vi "Demo7-Broader_Control_Panel.vi"() -> ()   [LabVIEW 2020]
panel:
  in  "Visualization Tab Control":enum32{"Trace", "Metrics"}(tab)
  out "Diode Trace":waveform(dbl)[](graph)
  out "Reduced Mean Signal, One Point = One Shot":dbl[](graph)
  out "(For your Reference: ) Query Sent to Device":string
  in  "Zero Time":bool
  out "Settable Device Keywords":string[](array[string])
  out "Live Readback Values":string[](array[string])
  in  "Set All":bool
  in  "Set Values\n(Fully empty cells will not be set)":string[](array[string])
  out "Live Responses":string[](array[string])
  out "Non-Settable Device Keywords":string[](array[string])
  in  "IP Address of Remote Device":string="196.254.31.200"
  in  "Disconnect":bool
  # "Diode Demo - General Purpose Control Panel"
  # "General control panel to facilitate setup of diode, setting times, verifying quality of metrics."
  # "VI Instructions\n\n1. Make sure you know the Device IP Address.\n2. From Windows command prompt, confirm ping to IP address.\n3. Type the correct device IP address into this VI.\n3. Run this VI. *Note:* Only one TCP connection to the device's SCPI-like server can run at a time.\n4. When finished, disconnect safely from the device via the \"Disconnect\" toggle button. (Not the Abort button).\n\nCreated by Scott Feister on July 19, 2022.\nUpdated back panel details July 28, 2022."
  # "1. Resets the trigger count to zero.\n2. Transmits this system's current time."
  # "Settings *ARE NOT SAVED TO DEVICE* and are lost on device reset! Write them down!"
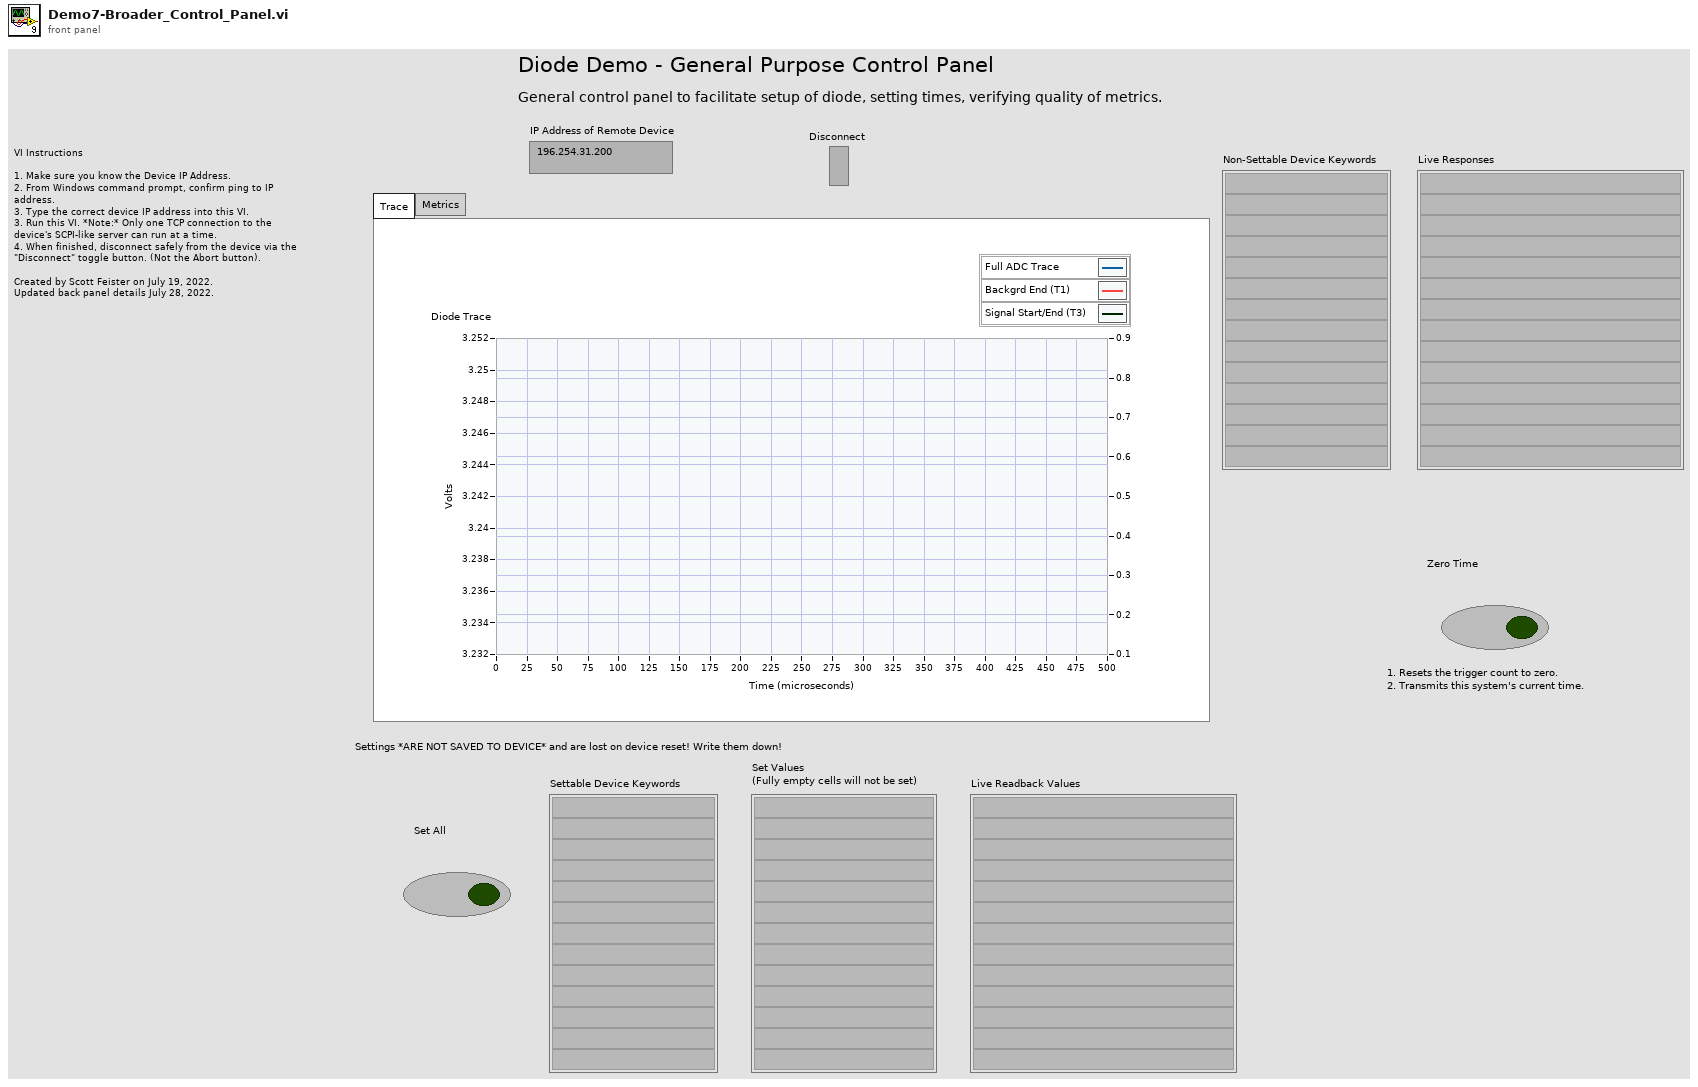
[diagram p1: front panel]
types:
  T1 = typedef "DDAQ-Keyword.ctl" = cluster{"Keyword":string, "Gettable":bool, "Settable":bool, "Is Array":bool, "Data Type":string, "Description":string}
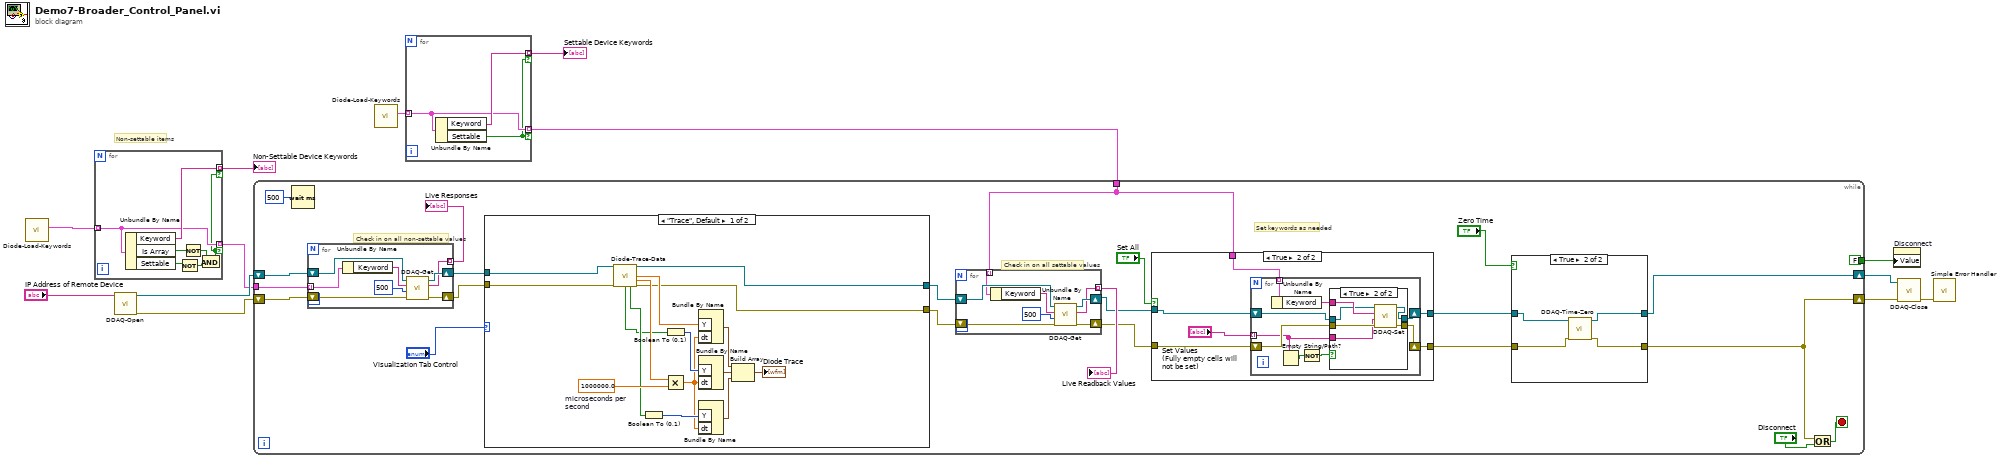
[diagram p0: block diagram]
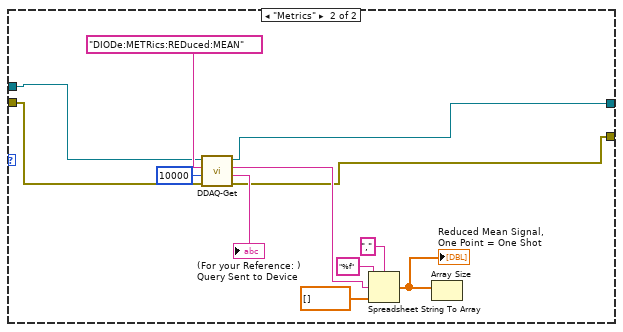
[diagram p2: hidden frame]
diagram:
  # "Non-settable items"
  n1 = call "Diode-Load-Keywords.vi"() -> ("Diodes Keywords Array"=w6:T1[])  [unwired: 11 in]
  n2 = for {
    tunnel: w6 -> [w18] mode=indexing
    tunnel: [w20] -> w5 mode=indexing if=w14
    tunnel: [w18] -> w4 mode=indexing if=w14
    n3 = Unbundle By Name(w18) -> ("Keyword"=w20:string, "Is Array"=w19:bool, "Settable"=w17:bool)
    n4 = Not(x=w17) -> (.not. x?=w16:bool)
    n5 = Not(x=w19) -> (.not. x?=w15:bool)
    n6 = And(x=w15, y=w16) -> (x .and. y?=w14:bool)
  }
  "Non-Settable Device Keywords" <- w5
  n7 = call "DDAQ-Open.vi"("IP Address of Nucleo Device"="IP Address of Remote Device") -> ("error out"=w12:errorcluster, "connection ID"=w13:refnum<k5>)  [unwired: 8 in, 1 out]
  n8 = call "Diode-Load-Keywords.vi"() -> ("Diodes Keywords Array"=w3:T1[])  [unwired: 11 in]
  n9 = for {
    tunnel: w3 -> [w22] mode=indexing
    tunnel: [w23] -> w2 mode=indexing if=w21
    tunnel: [w22] -> w1 mode=indexing if=w21
    n10 = Unbundle By Name(w22) -> ("Keyword"=w23:string, "Settable"=w21:bool)
  }
  "Settable Device Keywords" <- w2
  n11 = while {
    shift-right: [w26] -> w11
    shift-left: w13 -> [w46]
    shift-right: [w25] -> w10
    shift-left: w12 -> [w45]
    tunnel: [FALSE] -> w8
    tunnel: w4 -> [w39]
    tunnel: w1 -> [w32]
    stop <- w41 stop-if-true
    # "Set keywords as needed"
    # "Check in on all settable values"
    # "Check in on all non-settable values"
    n12 = Wait (ms)(milliseconds to wait=u32 500) -> ()  [unwired: 1 out]
    n13 = for {
      shift-right: [w119] -> w38
      shift-left: w46 -> [w121]
      shift-right: [w118] -> w37
      shift-left: w45 -> [w120]
      tunnel: [w116] -> w40 mode=indexing
      tunnel: w39 -> [w115] mode=indexing
      n14 = Unbundle By Name(w115) -> ("Keyword"=w114:string)
      n15 = call "DDAQ-Get.vi"("error in (no error)"=w120, "max bytes to read (10000)"=500 ("max bytes to read (500)"), "SCPI-like Keyword (leave off question mark)"=w114, "connection ID"=w121) -> ("error out"=w118:errorcluster, "Response"=w116:string, "connection ID out"=w119:refnum<k5>)  [unwired: 3 in, 2 out]
    }
    "Live Responses" <- w40
    n16 = case shown="\"Trace\", Default" "Visualization Tab Control" {
      tunnel: w38 -> [w62 w66]
      tunnel: w37 -> [w61 w65]
      tunnel: [w48 w63] -> w31
      tunnel: [w47 w64] -> w30
      frame "Trace", Default {
        w58 = 1000000.0  # microseconds per second
        n17 = call "Diode-Trace-Data.vi"("connection ID"=w62, "error in (no error)"=w61) -> ("connection ID out"=w48:refnum<k5>, "Trace (Volts)"=w60:dbl[], "dt"=w59:dbl, "Background Mask Array"=w49:bool[], "Signal Mask Array"=w50:bool[], "error out"=w47:errorcluster)  [unwired: 5 in, 3 out]
        n18 = Boolean To (0,1)(Boolean=w50) -> (0, 1=w56:i16[])
        n19 = Boolean To (0,1)(Boolean=w49) -> (0, 1=w57:i16[])
        n20 = Multiply(x=w59, y=w58) -> (x*y=w55:dbl)
        n21 = Bundle By Name("Y"=w60, "dt"=w55) -> (w52:waveform(dbl))  [unwired: 1 in]
        n22 = Bundle By Name("Y"=w57, "dt"=w55) -> (w54:waveform(i16))  [unwired: 1 in]
        n23 = Bundle By Name("Y"=w56, "dt"=w55) -> (w53:waveform(i16))  [unwired: 1 in]
        n24 = Build Array(w52, w54, w53) -> (→"Diode Trace":waveform(dbl)[])
      }
      frame "Metrics" {
        n25 = call "DDAQ-Get.vi"("error in (no error)"=w65, "max bytes to read (10000)"=10000 ("max bytes to read (500)"), "SCPI-like Keyword (leave off question mark)"="DIODe:METRics:REDuced:MEAN" ("Diode Keyword (leave off question mark)"), "connection ID"=w66) -> ("error out"=w64:errorcluster, "Query"=→"(For your Reference: ) Query Sent to Device":string, "Response"=w73:string, "connection ID out"=w63:refnum<k5>)  [unwired: 3 in, 1 out]
        n26 = Spreadsheet String To Array(delimiter (Tab)=",", format string="%f", spreadsheet string=w73, array type (2D Dbl)=dbl[] []) -> (array=w74:dbl[])
        "Reduced Mean Signal, One Point = One Shot" <- w74
        n27 = Array Size(array=w74) -> ()  [unwired: 1 out]
      }
    }
    n28 = for {
      shift-right: [w111] -> w34
      shift-left: w31 -> [w113]
      shift-right: [w110] -> w33
      shift-left: w30 -> [w112]
      tunnel: [w108] -> w36 mode=indexing
      tunnel: w32 -> [w107] mode=indexing
      n29 = Unbundle By Name(w107) -> ("Keyword"=w106:string)
      n30 = call "DDAQ-Get.vi"("error in (no error)"=w112, "max bytes to read (10000)"=500 ("max bytes to read (500)"), "SCPI-like Keyword (leave off question mark)"=w106, "connection ID"=w113) -> ("error out"=w110:errorcluster, "Response"=w108:string, "connection ID out"=w111:refnum<k5>)  [unwired: 3 in, 2 out]
    }
    "Live Readback Values" <- w36
    n31 = case shown="True" "Set All" {
      tunnel: w32 -> [_ w87]
      tunnel: w34 -> [w81 w86]
      tunnel: w33 -> [w82 w85]
      tunnel: [w82 w84] -> w27
      tunnel: [w81 w83] -> w28
      frame False {
      }
      frame True {
        n32 = for {
          tunnel: "Set Values\n(Fully empty cells will not be set)" -> [w89] mode=indexing
          tunnel: w87 -> [w97] mode=indexing
          shift-right: [w91] -> w84
          shift-left: w85 -> [w92]
          shift-right: [w90] -> w83
          shift-left: w86 -> [w95]
          n33 = Unbundle By Name(w97) -> ("Keyword"=w96:string)
          n34 = Empty String/Path?(string/path=w89) -> (empty?=w93:bool)
          n35 = Not(x=w93) -> (.not. x?=w94:bool)
          n36 = case shown="True" w94 {
            tunnel: w96 -> [_ w105]
            tunnel: w95 -> [w98 w104]
            tunnel: w92 -> [w99 w103]
            tunnel: [w99 w102] -> w91
            tunnel: [w98 w101] -> w90
            tunnel: w89 -> [_ w100]
            frame False {
            }
            frame True {
              n37 = call "DDAQ-Set.vi"("error in (no error)"=w103, "Set Value"=w100, "SCPI-like Keyword (leave off space, value)"=w105, "connection ID"=w104) -> ("error out"=w102:errorcluster, "connection ID out"=w101:refnum<k5>)  [unwired: 5 in, 1 out]
            }
          }
        }
      }
    }
    n38 = case shown="True" "Zero Time" {
      tunnel: w28 -> [w75 w80]
      tunnel: [w76 w77] -> w25
      tunnel: w27 -> [w76 w78]
      tunnel: [w75 w79] -> w26
      frame False {
      }
      frame True {
        n39 = call "DDAQ-Time-Zero.vi"("error in (no error)"=w78, "connection ID"=w80) -> ("error out"=w77:errorcluster, "connection ID out"=w79:refnum<k5>)  [unwired: 8 in]
      }
    }
    n40 = Or(x=w25, y="Disconnect") -> (x .or. y?=w41:bool)
  }
  n41 = property on="Disconnect" class="Bool (strict)"("Value"=w8) -> ()  [unwired: 2 in, 2 out]
  n42 = call "DDAQ-Close.vi"("error in (no error)"=w10, "connection ID"=w11) -> ("error out"=w9:errorcluster)  [unwired: 8 in, 1 out]
  n43 = call <vilib>:"Simple Error Handler.vi"("error in (no error)"=w9) -> ()  [unwired: 4 in, 5 out]
